vi "Example Instrument. Write Configuration.vi"(8 "error in (no error)":errorcluster, 10 "Configuration":T1, 11 "Example Instrument in":refnum<class "Example Instrument.lvclass">) -> (0 "error out":errorcluster, 3 "Example Instrument out":refnum<class "Example Instrument.lvclass">)   [LabVIEW 2016, in "Example Instrument.lvclass"]
uses:
  Example Instrument.lvclass
  Typedefs/Configuration--Cluster.ctl
  Example Instrument.lvclass/Example Instrument.ctl
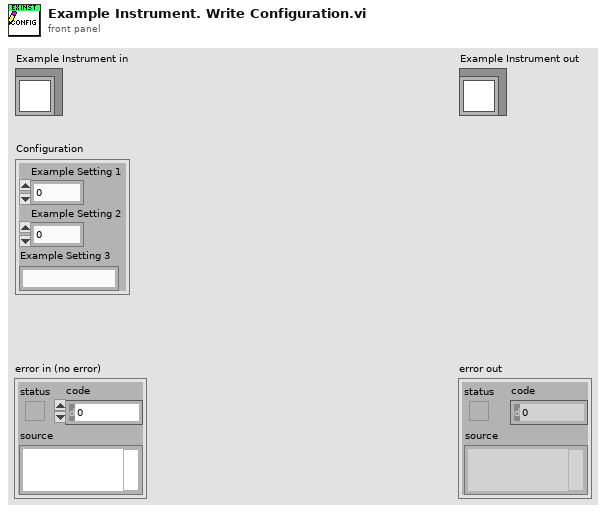
[diagram p1: front panel]
types:
  T1 = typedef "Example Instrument.lvclass/Configuration--Cluster.ctl" = cluster{"Example Setting 1":dbl, "Example Setting 2":dbl, "Example Setting 3":string}
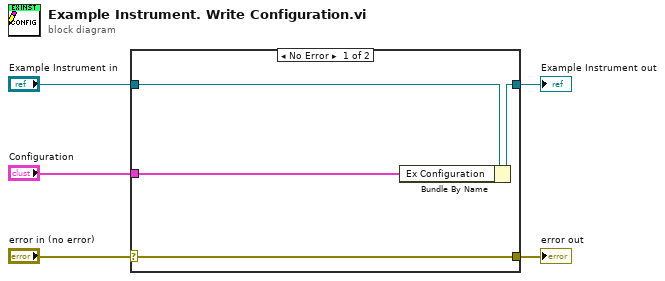
[diagram p0: block diagram]
diagram:
  n1 = case shown="No Error" "error in (no error)" {
    selector: "error in (no error)" -> [w9 w10]
    tunnel: [w9 w10] -> w4
    tunnel: [w7 w11] -> w2
    tunnel: "Example Instrument in" -> [w8 w11]
    tunnel: "Configuration" -> [w6 _]
    frame No Error {
      n2 = Bundle By Name(cluster=w8, "Ex Configuration"=w6) -> (w7:refnum<class "Example Instrument.lvclass">)
    }
    frame Error {
    }
  }
  "error out" <- w4
  "Example Instrument out" <- w2
